vi "Remove_Users_fr_Path.vi"(1 "File Path In":path) -> (0 "File Path Out":path)   [LabVIEW 2010]
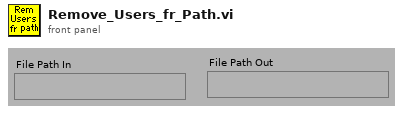
[diagram p1: front panel]
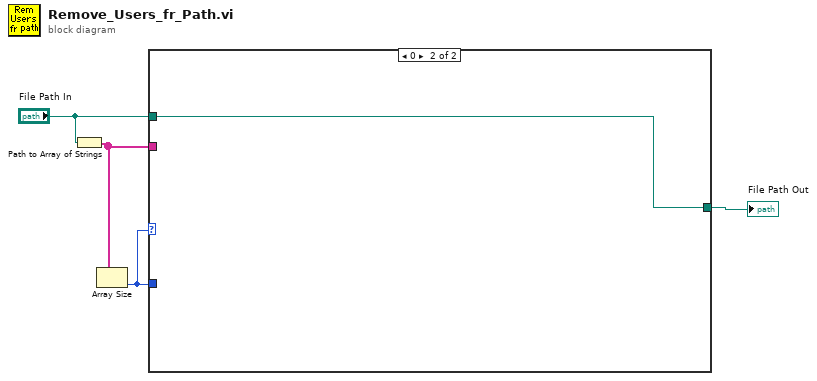
[diagram p0: block diagram]
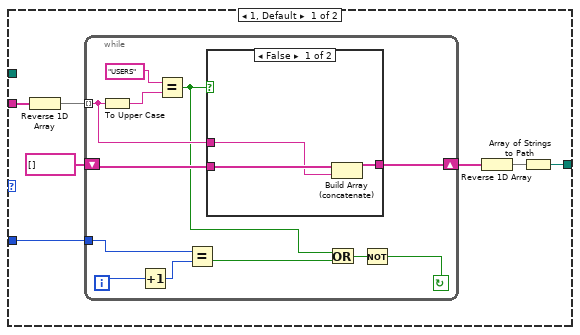
[diagram p2: hidden frame]
diagram:
  n1 = Path to Array of Strings(0:"File Path In") -> (2:w3:string[])  [unwired: 1 out]
  n2 = Array Size(array=w3) -> (size(s)=w2:i32)
  n3 = case shown="0" w2 {
    tunnel: [w10 w28] -> w4
    tunnel: w2 -> [w8 _]
    tunnel: w3 -> [w6 _]
    tunnel: "File Path In" -> [_ w28]
    frame 1, Default {
      n4 = Reverse 1D Array(array=w6) -> (reversed array=w5:string[])
      n5 = while {
        tunnel: w8 -> [w17]
        shift-left: string[] [] -> [w21]
        shift-right: [w20] -> w9
        tunnel: w5 -> [w19] mode=indexing
        i -> [w18]
        stop <- w12 continue-if-true
        n6 = To Upper Case(1:w19) -> (0:w23:string)
        n7 = Increment(x=w18) -> (x+1=w16:i32)
        n8 = Equal?(x="USERS", y=w23) -> (x = y?=w14:bool)
        n9 = Equal?(x=w17, y=w16) -> (x = y?=w15:bool)
        n10 = case shown="False" w14 {
          tunnel: w21 -> [w26 w27]
          tunnel: [w25 w27] -> w20
          tunnel: w19 -> [w24 _]
          frame False {
            n11 = Build Array (concatenate)(w26, w24) -> (w25:string[])
          }
          frame True {
          }
        }
        n12 = Or(x=w14, y=w15) -> (x .or. y?=w13:bool)
        n13 = Not(x=w13) -> (.not. x?=w12:bool)
      }
      n14 = Reverse 1D Array(array=w9) -> (reversed array=w11:string[])
      n15 = Array of Strings to Path(0:w11) -> (2:w10:path)  [unwired: 1 in]
    }
    frame 0 {
    }
  }
  "File Path Out" <- w4
